vi "Set Channel.vi"(8 "error in (no error)":errorcluster, 10 "Channel":T1, 11 "Optical Power Meter in":refnum<class "Optical Power Meter.lvclass">) -> (0 "error out":errorcluster, 3 "Optical Power Meter out":refnum<class "Optical Power Meter.lvclass">)   [LabVIEW 2018, in "Optical Power Meter.lvlib" / "Optical Power Meter.lvclass"]
uses:
  Optical Power Meter.lvclass
  Custom Controls/Channel List.ctl
  Optical Power Meter.lvlib
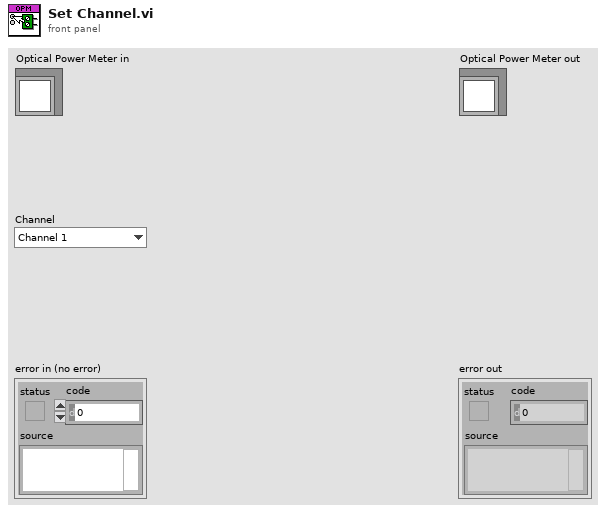
[diagram p1: front panel]
types:
  T1 = typedef "Optical Power Meter.lvlib/Channel List.ctl" = enum16{"Channel 1", "Channel 2", "Channel 3", "Channel 4"}
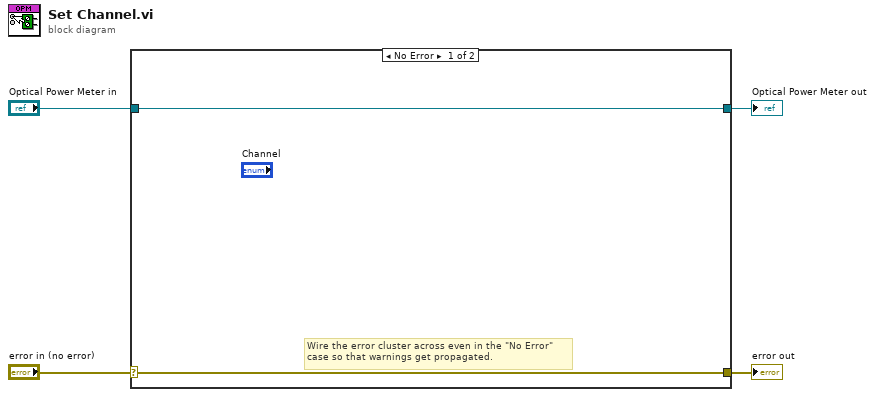
[diagram p0: block diagram]
diagram:
  n1 = case shown="No Error" "error in (no error)" {
    selector: "error in (no error)" -> [w5 w8]
    tunnel: [w5 w8] -> w3
    tunnel: [w6 w7] -> w1
    tunnel: "Optical Power Meter in" -> [w6 w7]
    frame No Error {
      # "Wire the error cluster across even in the \"No Error\"\ncase so that warnings get propagated."
    }
    frame Error {
    }
  }
  "error out" <- w3
  "Optical Power Meter out" <- w1
